vi "Set Default FP Background Color.vi"(8 "error in (no error)":errorcluster, 11 "vi path":path) -> (0 "error out":errorcluster)   [LabVIEW 2020]
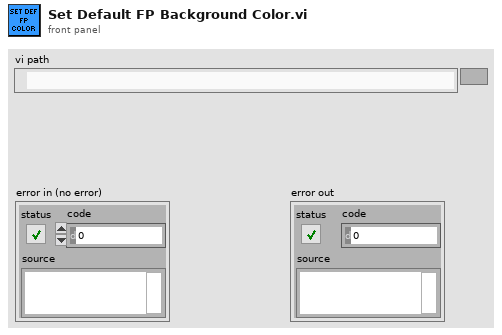
[diagram p1: front panel]
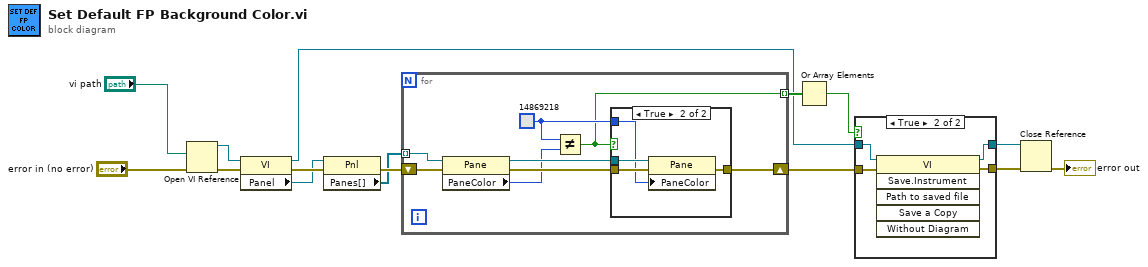
[diagram p0: block diagram]
diagram:
  n1 = Open VI Reference(vi path="vi path", error in (no error)="error in (no error)") -> (vi reference=w8:refnum<vi>, error out=w9:errorcluster)  [unwired: 4 in]
  n2 = property class="VI"(reference=w8, error in=w9) -> (reference out=w1:refnum<vi>, error out=w7:errorcluster, "Panel"=w6:refnum<vi>)
  n3 = property class="Pnl"(reference=w6, error in=w7) -> (error out=w5:errorcluster, "Panes[]"=w4:refnum<vi>[])  [unwired: 1 out]
  n4 = for {
    tunnel: w4 -> [w22] mode=indexing
    shift-right: [w17] -> w10
    shift-left: w5 -> [w23]
    tunnel: [w16] -> w3 mode=indexing
    w18 = u32 14869218
    n5 = property class="Pane"(reference=w22, error in=w23) -> (reference out=w20:refnum<vi>, error out=w21:errorcluster, "PaneColor"=w19:u32)
    n6 = Not Equal?(x=w18, y=w19) -> (x != y?=w16:bool)
    n7 = case shown="True" w16 {
      tunnel: w21 -> [w24 w28]
      tunnel: w20 -> [_ w27]
      tunnel: w18 -> [_ w26]
      tunnel: [w24 w25] -> w17
      frame False {
      }
      frame True {
        n8 = property class="Pane"(reference=w27, error in=w28, "PaneColor"=w26) -> (error out=w25:errorcluster)  [unwired: 1 out]
      }
    }
  }
  n9 = Or Array Elements(Boolean array=w3) -> (logical OR=w2:bool)
  n10 = case shown="True" w2 {
    tunnel: [w30 w34] -> w12
    tunnel: [w29 w33] -> w11
    tunnel: w10 -> [w30 w32]
    tunnel: w1 -> [w29 w31]
    frame False {
    }
    frame True {
      n11 = invoke class="VI" method="Save.Instrument"(reference=w31, error in=w32) -> (reference out=w33:refnum<vi>, error out=w34:errorcluster)  [unwired: 4 in, 4 out]
    }
  }
  n12 = Close Reference(reference=w11, error in (no error)=w12) -> (error out=→"error out":errorcluster)
